vi "voxel plot v2.vi"(4 "Update time":dbl, 5 "Map Data In":T1(array[cluster]), 6 "Sensor position":cluster{"X":sgl, "Y":sgl, "Z":sgl}={"X"=0.0, "Y"=0.0, "Z"=70.75}, 7 "Chunk length":u8=8, 8 "voxel length":dbl=8.0 format="%#_13g") -> (0 "error out":errorcluster, 3 "Scene":refnum<vi>)   [LabVIEW 2014]
uses:
  <vilib>/picture/3D Picture Control/Object/Create Object (name).vi
  <vilib>/picture/3D Picture Control/NI_3D Picture Control.lvlib
panel:
  out "object count":i32
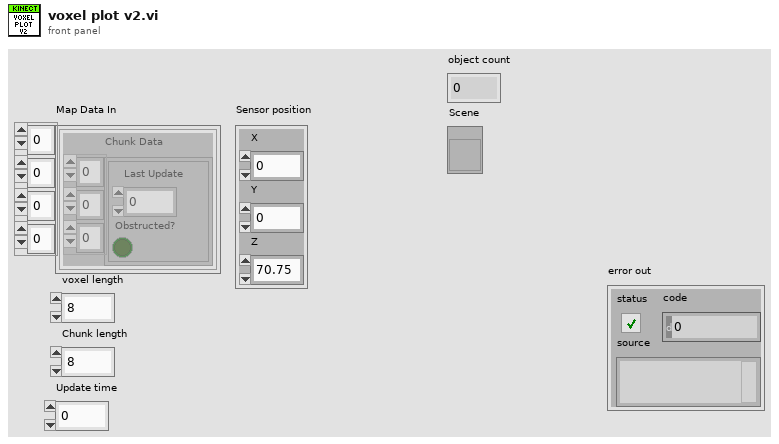
[diagram p1: front panel]
types:
  T1 = cluster{"Chunk Data":cluster{"Last Update":u32, "Obstructed?":bool}[][][]}[][][][]
  T2 = enum16{"Inherit Value", "Points", "Wireframe", "Polygons"}
  T3 = cluster{"Last Update":u32, "Obstructed?":bool}[][][]
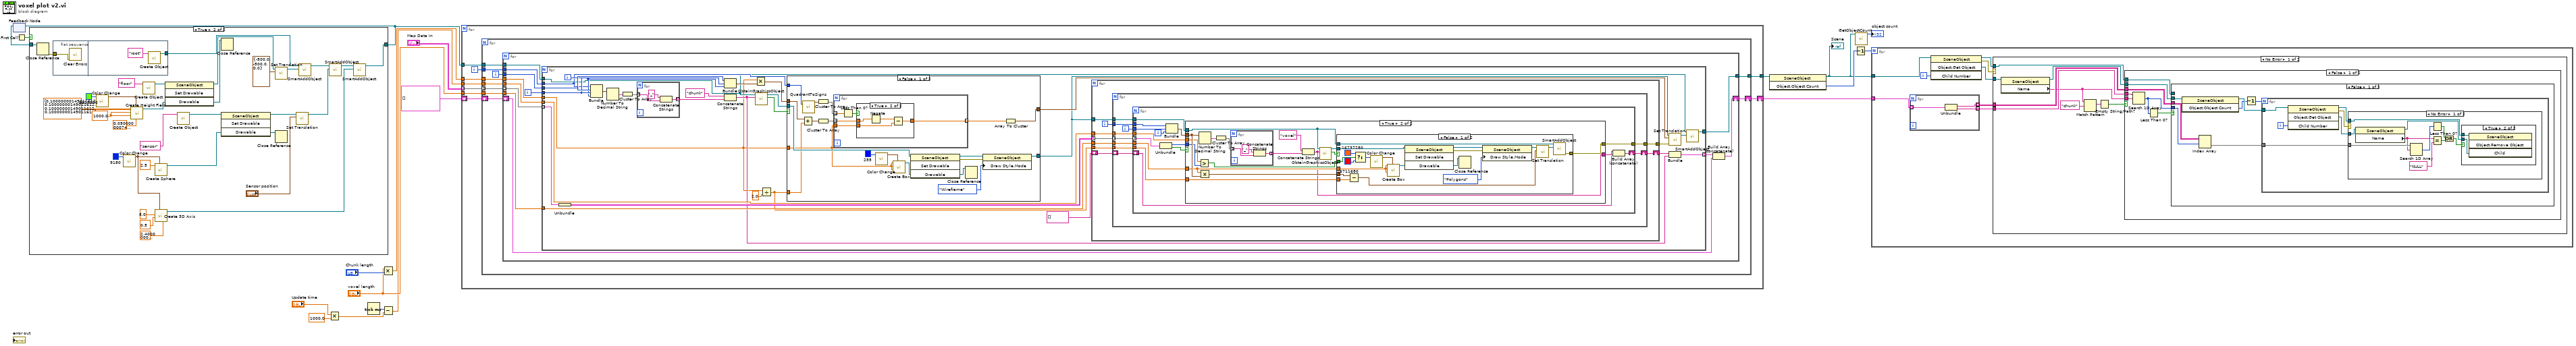
[diagram p0: block diagram]
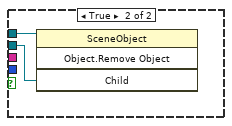
[diagram p5: hidden frame]
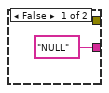
[diagram p8: hidden frame]
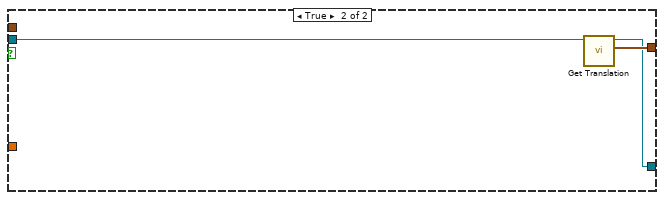
[diagram p11: hidden frame]
diagram:
  n1 = feedback #1() -> (w4:refnum<vi>)  [unwired: 1 in]
  n2 = First Call?() -> (First Call?: T/F=w1:bool)
  n3 = case shown="True" w1 {
    tunnel: [w20 w52] -> w7
    tunnel: w4 -> [w20 w22]
    frame False {
    }
    frame True {
      w49 = sgl 1000.0 ("Row Interval")
      n4 = Close Reference(reference=w22) -> (error out=w21:errorcluster)  [unwired: 1 in]
      n5 = flat-sequence {
        tunnel: w21 -> [w53]
        tunnel: [w54] -> w24
        frame #0 {
          n6 = call <vilib>:"Clear Errors.vi"("error in (no error)"=w53) -> ()  [unwired: 5 in, 2 out]
        }
        frame #1 {
          n7 = call-poly <vilib>:"Create Object.vi"("Name"="root") -> ("Scene:New Object"=w54:refnum<vi>)  [unwired: 9 in, 1 out]
        }
      }
      n8 = call <vilib>:"Color Change.vi"("Color"=u32 6618880) -> ("RGBA"=w47:cluster{"R":sgl, "G":sgl, "B":sgl, "A":sgl})  [unwired: 10 in]
      n9 = call <vilib>:"Color Change.vi"("Color"=u32 9180) -> ("RGBA"=w29:cluster{"R":sgl, "G":sgl, "B":sgl, "A":sgl})  [unwired: 10 in]
      n10 = call <vilib>:"Create Height Field.vi"("Base Height"=sgl 0.05, "Color"=w47, "Column Interval"=w49, "Row Interval"=w49, "Data"=sgl[][] [[0.1, 0.1], [0.1, 0.1]]) -> ("New Height Field Refnum"=w44:refnum<vi>)  [unwired: 5 in, 1 out]
      n11 = call-poly <vilib>:"Create Object.vi"("Name"="floor") -> ("Scene:New Object"=w45:refnum<vi>)  [unwired: 9 in, 1 out]
      n12 = call <vilib>:"Create Sphere.vi"("Color"=w29, "Radius"=sgl 2.5) -> ("New Sphere Refnum"=w34:refnum<vi>)  [unwired: 8 in, 1 out]
      n13 = call <vilib>:"Create 3D Axis.vi"("Character Size"=sgl 2.4, "Color"=w29, "Radius"=sgl 0.5, "Length"=sgl 8.0) -> ("New Object Refnum"=w28:refnum<vi>)  [unwired: 6 in, 1 out]
      n14 = invoke class="SceneObject" method="Set Drawable"(reference=w45, "Drawable"=w44) -> (reference out=w42:refnum<vi>, "Drawable"=w43:refnum<vi>)  [unwired: 2 in, 2 out]
      n15 = call-poly <vilib>:"Create Object.vi"("Name"="sensor") -> ("Scene:New Object"=w39:refnum<vi>)  [unwired: 9 in, 1 out]
      n16 = Close Reference(reference=w43) -> ()  [unwired: 1 in, 1 out]
      n17 = invoke class="SceneObject" method="Set Drawable"(reference=w39, "Drawable"=w34) -> (reference out=w38:refnum<vi>, "Drawable"=w33:refnum<vi>)  [unwired: 2 in, 2 out]
      n18 = call <vilib>:"Set Translation.vi"("Translation"=cluster{"X":sgl, "Y":sgl, "Z":sgl} {"X"=-500.0, "Y"=-500.0, "Z"=0.0}, "Scene Object"=w42) -> ("Translated Object"=w26:refnum<vi>)  [unwired: 8 in, 1 out]
      n19 = Close Reference(reference=w33) -> ()  [unwired: 1 in, 1 out]
      n20 = call <vilib>:"Set Translation.vi"("Translation"="Sensor position", "Scene Object"=w38) -> ("Translated Object"=w27:refnum<vi>)  [unwired: 8 in, 1 out]
      n21 = call "SmartAddObject.vi"("New Object In"=w26, "Scene Object In"=w24) -> ("Scene Object Out"=w25:refnum<vi>)  [unwired: 8 in, 1 out]
      n22 = call "SmartAddObject.vi"("New Object In"=w27, "Scene Object In"=w25) -> ("Scene Object Out"=w23:refnum<vi>)  [unwired: 8 in, 1 out]
      n23 = call "SmartAddObject.vi"("New Object In"=w28, "Scene Object In"=w23) -> ("Scene Object Out"=w52:refnum<vi>)  [unwired: 8 in, 1 out]
    }
  }
  n24 = feedback-in #1(w7) -> ()
  n25 = Multiply(x="Update time", y=1000.0) -> (x*y=w13:dbl)
  n26 = Tick Count (ms)() -> (millisecond timer value=w12:u32)
  n27 = Multiply(x="voxel length", y="Chunk length") -> (x*y=w17:dbl)
  n28 = Subtract(x=w12, y=w13) -> (x-y=w11:dbl)
  n29 = for {
    tunnel: "Map Data In" -> [w64] mode=indexing
    tunnel: w7 -> [w62]
    tunnel: w17 -> [w61]
    tunnel: "voxel length" -> [w60]
    tunnel: w11 -> [w59]
    tunnel: [w58] -> w9
    shift-right: [w56] -> w8
    shift-left: cluster{string[], string}[] [] -> [w57]
    i -> [w63]
    n30 = for {
      tunnel: w64 -> [w74] mode=indexing
      tunnel: w63 -> [w73]
      tunnel: w62 -> [w71]
      tunnel: w61 -> [w70]
      tunnel: w60 -> [w69]
      tunnel: w59 -> [w68]
      tunnel: [w67] -> w58
      shift-right: [w65] -> w56
      shift-left: w57 -> [w66]
      i -> [w72]
      n31 = for {
        tunnel: w74 -> [w86] mode=indexing
        tunnel: w73 -> [w85]
        tunnel: w72 -> [w84]
        tunnel: w71 -> [w82]
        tunnel: w70 -> [w81]
        tunnel: w69 -> [w80]
        tunnel: w68 -> [w79]
        tunnel: [w78] -> w67
        shift-right: [w76] -> w65
        shift-left: w66 -> [w75]
        i -> [w83]
        n32 = for {
          tunnel: w86 -> [w103] mode=indexing
          tunnel: w85 -> [w104]
          tunnel: w84 -> [w111]
          tunnel: w83 -> [w110]
          tunnel: w82 -> [w97]
          tunnel: w81 -> [w89]
          tunnel: w80 -> [w101]
          tunnel: w79 -> [w100]
          tunnel: [w96] -> w78
          tunnel: [w92] -> w77 mode=indexing
          i -> [w109]
          n33 = Unbundle(w103) -> ("Chunk Data"=w102:T3)
          n34 = Bundle(w104, w111, w110, w109) -> (w112:cluster{i32, i32, i32, i32})  [unwired: 1 in]
          n35 = Number To Decimal String(number=w112) -> (decimal integer string=w116:cluster{string, string, string, string})  [unwired: 1 in]
          n36 = Cluster To Array(cluster=w116) -> (array=w115:string[])
          n37 = for {
            tunnel: w115 -> [w224] mode=indexing
            tunnel: [w222] -> w113 mode=indexing
            n38 = Concatenate Strings("_" ("string"), w224) -> (w222:string)
          }
          n39 = Bundle(w111, w110, w109) -> (w108:cluster{i32, i32, i32})  [unwired: 1 in]
          n40 = Concatenate Strings("chunk" ("string"), w113) -> (w93:string)
          n41 = Multiply(x=w89, y=w108) -> (x*y=w105:cluster{dbl, dbl, dbl})
          n42 = call "ObtainGraphicsObject.vi"("Object Name"=w93, "Scene in"=w97) -> ("Found?"=w107:bool, "Scene:New Object"=w106:refnum<vi>)  [unwired: 8 in]
          n43 = Divide(x=w89, y=2.0) -> (x/y=w87:dbl)
          n44 = case shown="False" w107 {
            tunnel: w106 -> [w208 w221]
            tunnel: w89 -> [w197 _]
            tunnel: w105 -> [w192 _]
            tunnel: w104 -> [w196 _]
            tunnel: [w195 w220] -> w99
            tunnel: [w194 w219] -> w90
            tunnel: w87 -> [w190 _]
            frame False {
              n45 = Add(x=w192, y=w190) -> (x+y=w191:cluster{dbl, dbl, dbl})
              n46 = call "QuadrantToSigns.vi"("Quadrant"=w196) -> ("Point Out"=w198:cluster{"X":sgl, "Y":sgl, "Z":sgl})  [unwired: 18 in]
              n47 = Cluster To Array(cluster=w198) -> (array=w199:sgl[])
              n48 = Cluster To Array(cluster=w191) -> (array=w193:dbl[])
              n49 = for {
                tunnel: w199 -> [w209] mode=indexing
                tunnel: w197 -> [w212]
                tunnel: [w211] -> w200 mode=indexing
                tunnel: w193 -> [w210] mode=indexing
                n50 = Less Than 0?(x=w209) -> (x < 0?=w213:bool)
                n51 = case shown="True" w213 {
                  tunnel: w210 -> [w214 w216]
                  tunnel: w212 -> [_ w218]
                  tunnel: [w214 w217] -> w211
                  frame False {
                  }
                  frame True {
                    n52 = Negate(x=w216) -> (-x=w215:dbl)
                    n53 = Subtract(x=w215, y=w218) -> (x-y=w217:dbl)
                  }
                }
              }
              n54 = call <vilib>:"Color Change.vi"("Color"=u32 255) -> ("RGBA"=w202:cluster{"R":sgl, "G":sgl, "B":sgl, "A":sgl})  [unwired: 10 in]
              n55 = call <vilib>:"Create Box.vi"("Color"=w202, "Length Z"=w197, "Length Y"=w197, "Length X"=w197) -> ("New Box Refnum"=w201:refnum<vi>)  [unwired: 6 in, 1 out]
              n56 = invoke class="SceneObject" method="Set Drawable"(reference=w208, "Drawable"=w201) -> (reference out=w206:refnum<vi>, error out=w205:errorcluster, "Drawable"=w207:refnum<vi>)  [unwired: 2 in, 1 out]
              n57 = Close Reference(reference=w207) -> ()  [unwired: 1 in, 1 out]
              n58 = property class="SceneObject"(reference=w206, error in=w205, "Draw Style.Mode"=T2."Wireframe" ("Draw Style:Mode")) -> (reference out=w194:refnum<vi>)  [unwired: 1 out]
              n59 = Array To Cluster(array=w200) -> (cluster=w195:cluster{"[0]":dbl, "[1]":dbl, "[2]":dbl})
            }
            frame True {
              n60 = call <vilib>:"Get Translation.vi"("Scene Object"=w221) -> ("Transformation:Get Translation"=w220:cluster{"X":sgl, "Y":sgl, "Z":sgl}, "Scene Object"=w219:refnum<vi>)  [unwired: 8 in, 1 out]
            }
          }
          n61 = for {
            tunnel: w102 -> [w125] mode=indexing
            tunnel: w90 -> [w124]
            tunnel: w101 -> [w123]
            tunnel: w100 -> [w121]
            shift-right: [w120] -> w94
            shift-left: string[] [] -> [w119]
            tunnel: [w118] -> w91
            tunnel: w87 -> [w117]
            i -> [w122]
            n62 = for {
              tunnel: w125 -> [w135] mode=indexing
              tunnel: w124 -> [w134]
              tunnel: w123 -> [w133]
              tunnel: w122 -> [w131]
              tunnel: w121 -> [w130]
              shift-right: [w129] -> w120
              shift-left: w119 -> [w128]
              tunnel: [w127] -> w118
              tunnel: w117 -> [w126]
              i -> [w132]
              n63 = for {
                tunnel: w135 -> [w144] mode=indexing
                tunnel: w134 -> [w150]
                tunnel: w133 -> [w145]
                tunnel: w132 -> [w148]
                tunnel: w131 -> [w147]
                tunnel: w130 -> [w141]
                shift-right: [w139] -> w129
                shift-left: w128 -> [w138]
                tunnel: [w137] -> w127
                tunnel: w126 -> [w136]
                i -> [w149]
                n64 = Unbundle(w144) -> ("Last Update"=w142:u32, "Obstructed?"=w143:bool)
                n65 = Bundle(w147, w148, w149) -> (w146:cluster{i32, i32, i32})  [unwired: 1 in]
                n66 = case shown="True" w143 {
                  tunnel: w150 -> [_ w155]
                  tunnel: w146 -> [_ w163]
                  tunnel: w145 -> [_ w159]
                  tunnel: w142 -> [_ w157]
                  tunnel: w141 -> [_ w158]
                  tunnel: ["NULL" w154] -> w140
                  tunnel: [_ w153] -> w137
                  tunnel: w136 -> [_ w152]
                  frame False {
                  }
                  frame True {
                    n67 = Greater?(x=w158, y=w157) -> (0:w156:bool)
                    n68 = Multiply(x=w159, y=w163) -> (x*y=w161:cluster{dbl, dbl, dbl})
                    n69 = Number To Decimal String(number=w163) -> (decimal integer string=w167:cluster{string, string, string})  [unwired: 1 in]
                    n70 = Cluster To Array(cluster=w167) -> (array=w166:string[])
                    n71 = for {
                      tunnel: w166 -> [w189] mode=indexing
                      tunnel: [w187] -> w164 mode=indexing
                      n72 = Concatenate Strings("_" ("string"), w189) -> (w187:string)
                    }
                    n73 = Concatenate Strings("voxel" ("string"), w164) -> (w154:string)
                    n74 = call "ObtainGraphicsObject.vi"("Object Name"=w154, "Scene in"=w155) -> ("Found?"=w162:bool, "Scene:New Object"=w160:refnum<vi>)  [unwired: 8 in]
                    n75 = case shown="False" w162 {
                      tunnel: w161 -> [w170 _]
                      tunnel: w160 -> [w184 _]
                      tunnel: w159 -> [w185 _]
                      tunnel: w156 -> [w174 _]
                      tunnel: w155 -> [w172 _]
                      tunnel: [w171 _] -> w153
                      tunnel: w152 -> [w168 _]
                      frame False {
                        n76 = Subtract(x=w170, y=w168) -> (x-y=w169:cluster{dbl, dbl, dbl})
                        n77 = Select(t=u32 16737280 ("Color"), s=w174, f=u32 16711680 ("Color")) -> (s? t:f=w177:u32)
                        n78 = call <vilib>:"Color Change.vi"("Color"=w177) -> ("RGBA"=w186:cluster{"R":sgl, "G":sgl, "B":sgl, "A":sgl})  [unwired: 10 in]
                        n79 = call <vilib>:"Create Box.vi"("Color"=w186, "Length Z"=w185, "Length Y"=w185, "Length X"=w185) -> ("New Box Refnum"=w183:refnum<vi>)  [unwired: 6 in, 1 out]
                        n80 = invoke class="SceneObject" method="Set Drawable"(reference=w184, "Drawable"=w183) -> (reference out=w182:refnum<vi>, error out=w181:errorcluster, "Drawable"=w179:refnum<vi>)  [unwired: 2 in, 1 out]
                        n81 = Close Reference(reference=w179) -> ()  [unwired: 1 in, 1 out]
                        n82 = property class="SceneObject"(reference=w182, error in=w181, "Draw Style.Mode"=T2."Polygons" ("Draw Style:Mode")) -> (reference out=w178:refnum<vi>)  [unwired: 1 out]
                        n83 = call <vilib>:"Set Translation.vi"("Translation"=w169, "Scene Object"=w178) -> ("Translated Object"=w173:refnum<vi>)  [unwired: 8 in, 1 out]
                        n84 = call "SmartAddObject.vi"("New Object In"=w173, "Scene Object In"=w172) -> ("error out"=w171:errorcluster)  [unwired: 8 in, 1 out]
                      }
                      frame True {
                      }
                    }
                  }
                }
                n85 = Build Array (concatenate)(w138, w140) -> (w139:string[])
              }
            }
          }
          n86 = call <vilib>:"Set Translation.vi"("error in (no error)"=w91, "Translation"=w99, "Scene Object"=w90) -> ("Translated Object"=w98:refnum<vi>)  [unwired: 7 in, 1 out]
          n87 = Bundle(w94, w93) -> (w92:cluster{string[], string})  [unwired: 1 in]
          n88 = call "SmartAddObject.vi"("New Object In"=w98, "Scene Object In"=w97) -> ("Scene Object Out"=w96:refnum<vi>)  [unwired: 8 in, 1 out]
        }
        n89 = Build Array (concatenate)(w77, w75) -> (w76:cluster{string[], string}[])
      }
    }
  }
  n90 = invoke class="SceneObject" method="Object.Object Count"(reference=w9) -> (reference out=w3:refnum<vi>, "Child Count"=w5:i32)  [unwired: 2 in, 1 out]
  "Scene" <- w3
  n91 = Decrement(x=w5) -> (x-1=w6:i32)
  n92 = call "GetObjectCount.vi"("Scene Object In"=w3) -> ("object count"=→"object count":i32)  [unwired: 9 in, 1 out]
  n93 = for {
    N: w6 -> [_]
    tunnel: w3 -> [w231]
    tunnel: w8 -> [w229]
    i -> [w232]
    n94 = for {
      tunnel: w229 -> [w278] mode=indexing
      tunnel: [w277] -> w228 mode=indexing
      tunnel: [w276] -> w227 mode=indexing
      n95 = Unbundle(w278) -> (w276:string[], w277:string)
    }
    n96 = invoke class="SceneObject" method="Object.Get Object"(reference=w231, "Child Number"=w232) -> (reference out=w226:refnum<vi>, error out=w225:errorcluster, "Get Child"=w230:refnum<vi>)  [unwired: 2 in, 1 out]
    n97 = case shown="No Error" w225 {
      tunnel: w230 -> [w241 _]
      tunnel: w228 -> [w240 _]
      tunnel: w227 -> [w238 _]
      tunnel: w226 -> [w237 _]
      frame No Error {
        n98 = property class="SceneObject"(reference=w241) -> (reference out=w239:refnum<vi>, "Name"=w236:string)  [unwired: 1 in, 1 out]
        n99 = Match Pattern(string=w236, regular expression="chunk") -> (match substring=w234:string)  [unwired: 1 in, 3 out]
        n100 = Empty String/Path?(string/path=w234) -> (empty?=w233:bool)
        n101 = case shown="False" w233 {
          tunnel: w240 -> [w248 _]
          tunnel: w239 -> [w247 _]
          tunnel: w238 -> [w246 _]
          tunnel: w237 -> [w244 _]
          tunnel: w236 -> [w243 _]
          frame False {
            n102 = Search 1D Array(1D array=w248, element=w243) -> (index of element=w245:i32)  [unwired: 1 in]
            n103 = Less Than 0?(x=w245) -> (x < 0?=w242:bool)
            n104 = case shown="False" w242 {
              tunnel: w247 -> [w253 w275]
              tunnel: w244 -> [_ w274]
              tunnel: w246 -> [w255 _]
              tunnel: w245 -> [w254 _]
              frame False {
                n105 = invoke class="SceneObject" method="Object.Object Count"(reference=w253) -> (reference out=w251:refnum<vi>, "Child Count"=w250:i32)  [unwired: 2 in, 1 out]
                n106 = Index Array(array=w255, index (row)=w254) -> (element=w252:string[])  [unwired: 1 in]
                n107 = Decrement(x=w250) -> (x-1=w249:i32)
                n108 = for {
                  N: w249 -> [_]
                  tunnel: w252 -> [w258]
                  tunnel: w251 -> [w261]
                  i -> [w260]
                  n109 = invoke class="SceneObject" method="Object.Get Object"(reference=w261, "Child Number"=w260) -> (reference out=w257:refnum<vi>, error out=w256:errorcluster, "Get Child"=w259:refnum<vi>)  [unwired: 2 in, 1 out]
                  n110 = case shown="No Error" w256 {
                    tunnel: w259 -> [w271 _]
                    tunnel: w258 -> [w270 _]
                    tunnel: w257 -> [w267 _]
                    frame No Error {
                      n111 = property class="SceneObject"(reference=w271) -> (reference out=w268:refnum<vi>, "Name"=w264:string)  [unwired: 1 in, 1 out]
                      n112 = Search 1D Array(1D array=w270, element=w264) -> (index of element=w269:i32)  [unwired: 1 in]
                      n113 = Less Than 0?(x=w269) -> (x < 0?=w266:bool)
                      n114 = Equal?(x=w264, y="NULL") -> (x = y?=w263:bool)
                      n115 = Or(x=w266, y=w263) -> (x .or. y?=w265:bool)
                      n116 = case shown="True" w265 {
                        tunnel: w268 -> [_ w273]
                        tunnel: w267 -> [_ w272]
                        frame False {
                        }
                        frame True {
                          n117 = invoke class="SceneObject" method="Object.Remove Object"(reference=w272, "Child"=w273) -> ()  [unwired: 2 in, 4 out]
                        }
                      }
                    }
                    frame Error {
                    }
                  }
                }
              }
              frame True {
                n118 = invoke class="SceneObject" method="Object.Remove Object"(reference=w274, "Child"=w275) -> ()  [unwired: 2 in, 4 out]
              }
            }
          }
          frame True {
          }
        }
      }
      frame Error {
      }
    }
  }
